vi "createGUIEvent.vi"(8 "error in (no error)":errorcluster, 10 "event data":T1, 11 "User Event in":refnum<user-event>) -> (0 "error out":errorcluster)   [LabVIEW 2020]
uses:
  Controls/eventtypdef1.ctl
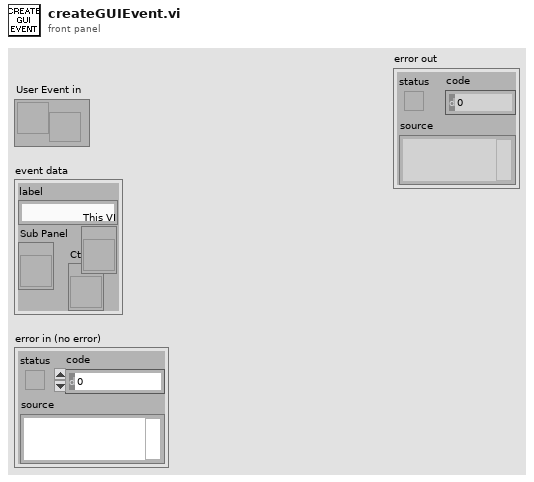
[diagram p1: front panel]
types:
  T1 = typedef "eventtypdef1.ctl" = cluster{"label":string, "Sub Panel":refnum<vi>, "CtlRef":refnum<vi>, "This VI":refnum<vi>}
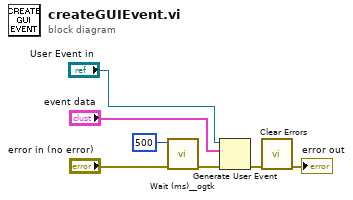
[diagram p0: block diagram]
diagram:
  n1 = call <userlib>:"Wait (ms)__ogtk.vi"("error in (no error)"="error in (no error)", "milliseconds to wait"=u32 500) -> ("error out"=w3:errorcluster)  [unwired: 8 in, 1 out]
  n2 = Generate User Event(user event="User Event in", event data cluster="event data", error in=w3) -> (error out=w4:errorcluster)  [unwired: 1 in, 1 out]
  n3 = call <vilib>:"Clear Errors.vi"("error in (no error)"=w4) -> ("error out"=→"error out":errorcluster)  [unwired: 5 in, 1 out]
